vi "COMI AD Get Volt.vi"(10 "ch":i32, 11 "hDevice":u32) -> (2 "function return":sgl, 3 "hDevice out":u32)   [LabVIEW 2017, in "Comidll.lvlib"]
doc: "float (COMI_AD_GetVolt) (HANDLE hDevice, int ch);"
uses:
  <userlib>/Comidll/Comidll.lvlib
  <userlib>/Comidll/Comidll.dll
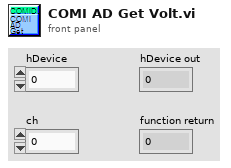
[diagram p1: front panel]
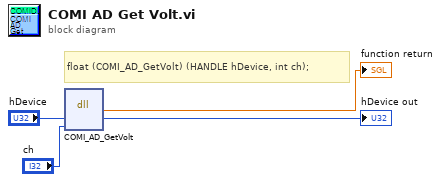
[diagram p0: block diagram]
diagram:
  # "float\t(COMI_AD_GetVolt) (HANDLE hDevice, int ch);"
  n1 = dll-call lib="C:/Program Files/National Instruments/LabVIEW 2017/user.lib/Comidll/Comidll.*" fn="COMI_AD_GetVolt"("hDevice"="hDevice", "ch"="ch") -> (→"function return":sgl, "hDevice"=→"hDevice out":u32)  [unwired: 4 in, 2 out]
